vi "LM Lorentzian and gradient.vi"(3 "output control":T1, 4 "data":variant, 5 "X":dbl[](array[numeric]), 6 "a":dbl[](array[numeric])) -> (0 "error out":errorcluster, 1 "f'(X,a)":dbl[][](array[numeric]), 2 "f(X,a)":dbl[](array[numeric]))   [LabVIEW 2019]
doc: "This template is the starting point for creating a model function to be passed to the Nonlinear Curve Fit.vi."
uses:
  <vilib>/gmath/NumericalOptimization/LM_output select.ctl
  <vilib>/gmath/NI_Gmath.lvlib
panel:
  # "Parameters:\n\namplitude: A\ncenter: t_0\nFWHM: w"
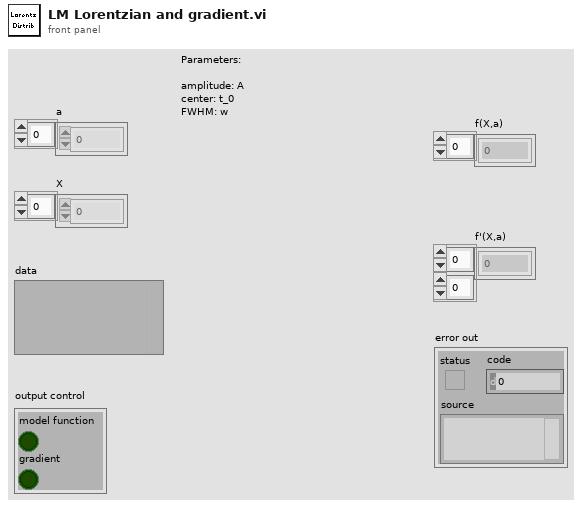
[diagram p1: front panel]
types:
  T1 = typedef "NI_Gmath.lvlib/LM_output select.ctl" = cluster{"model function":bool, "gradient":bool}
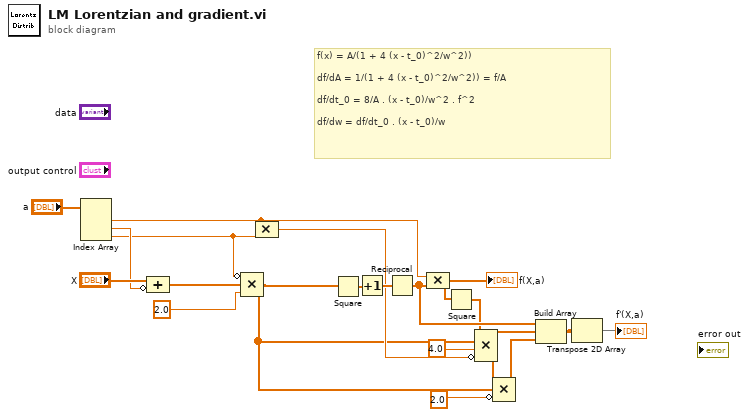
[diagram p0: block diagram]
diagram:
  # "f(x) = A/(1 + 4 (x - t_0)^2/w^2))\n\ndf/dA = 1/(1 + 4 (x - t_0)^2/w^2)) = f/A\n\ndf/dt_0 = 8/A . (x - t_0)/w^2 . f^2\n\ndf/dw = df/dt_0 . (x - t_0)/w"
  n1 = Index Array(array="a") -> (element #1=w7:dbl, element #2=w18:dbl, element #3=w8:dbl)  [unwired: 3 in]
  n2 = Compound Arithmetic op=ADD("X", invert w18) -> (w17:dbl[])
  n3 = Compound Arithmetic op=MULTIPLY(invert w8, w17, 2.0 ("element")) -> (w3:dbl[])
  n4 = Compound Arithmetic op=MULTIPLY(w7, w8) -> (w6:dbl)
  n5 = Square(x=w3) -> (x^2=w15:dbl[])
  n6 = Increment(x=w15) -> (x+1=w14:dbl[])
  n7 = Reciprocal(x=w14) -> (1/x=w13:dbl[])
  n8 = Compound Arithmetic op=MULTIPLY(w7, w13) -> (w10:dbl[])
  "f(X,a)" <- w10
  n9 = Square(x=w10) -> (x^2=w9:dbl[])
  n10 = Compound Arithmetic op=MULTIPLY(w9, w3, 4.0 ("result"), invert w6) -> (w4:dbl[])
  n11 = Compound Arithmetic op=MULTIPLY(w4, w3, invert 2.0 ("result")) -> (w1:dbl[])
  n12 = Build Array(w13, w4, w1) -> (w12:dbl[][])
  n13 = Transpose 2D Array(2D array=w12) -> (transposed array=→"f'(X,a)":dbl[][])
